vi "Joystick 2 LiftSystem.vi"(10 "Secondary Joystick Buttons":bool[](array[boolean]), 11 "JoystickAxes":dbl[](array[numeric])) -> (3 "Lift System Actions":T1)   [LabVIEW 2019]
uses:
  Controls/Lift System Actions.ctl
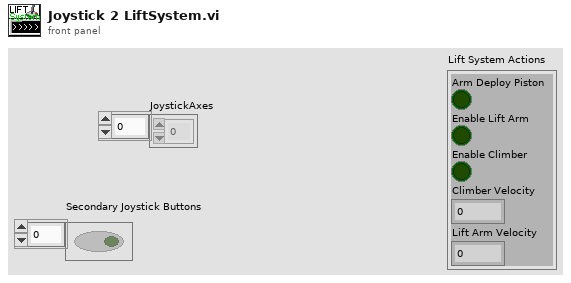
[diagram p1: front panel]
types:
  T1 = typedef "Lift System Actions.ctl" = cluster{"Arm Deploy Piston":bool, "Enable Lift Arm":bool, "Enable Climber":bool, "Climber Velocity":dbl, "Lift Arm Velocity":dbl}
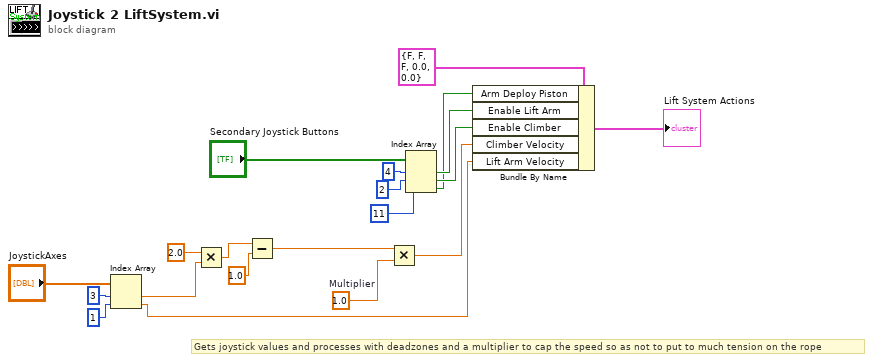
[diagram p0: block diagram]
diagram:
  w18 = 1.0  # Multiplier
  # "Gets joystick values and processes with deadzones and a multiplier to cap the speed so as not to put to much tension on the rope"
  n1 = Index Array(array="JoystickAxes", index #1=3 ("index"), index #2=1 ("index")) -> (element #1=w5:dbl, element #2=w13:dbl)
  n2 = Multiply(x=2.0, y=w5) -> (x*y=w3:dbl)
  n3 = Subtract(x=w3, y=1.0) -> (x-y=w1:dbl)
  n4 = Multiply(x=w1, y=w18) -> (x*y=w15:dbl)
  n5 = Index Array(array="Secondary Joystick Buttons", index #1=4 ("index"), index #2=2 ("index"), index #3=11 ("index")) -> (element #1=w9:bool, element #2=w8:bool, element #3=w6:bool)
  n6 = Bundle By Name(cluster=T1 {"Arm Deploy Piston"=FALSE, "Enable Lift Arm"=FALSE, "Enable Climber"=FALSE, "Climber Velocity"=0.0, "Lift Arm Velocity"=0.0} ("Lift System Actions"), "Arm Deploy Piston"=w6, "Enable Lift Arm"=w9, "Enable Climber"=w8, "Climber Velocity"=w15, "Lift Arm Velocity"=w13) -> (→"Lift System Actions":T1)
